vi "字符串解包.vi"(10 "输入数据":string, 11 "初始化缓存":i32[][](array[numeric])) -> (2 "解析后数据":i32[][](array[numeric]))   [LabVIEW 2020]
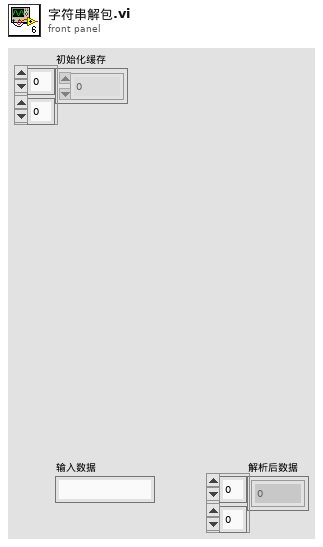
[diagram p1: front panel]
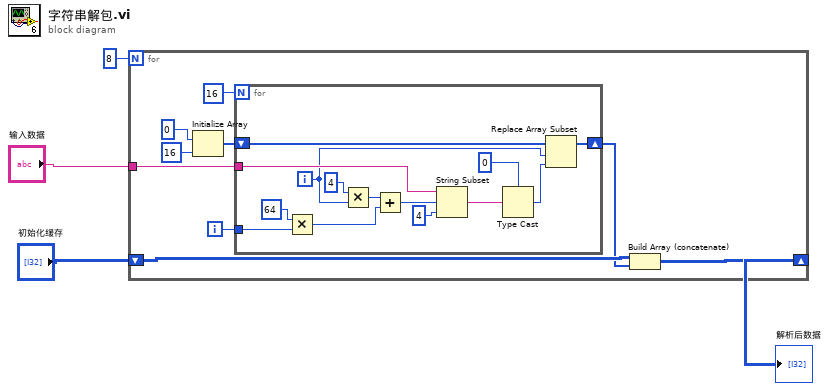
[diagram p0: block diagram]
diagram:
  n1 = for {
    N: u16 8 -> [_]
    tunnel: "输入数据" -> [w13]
    shift-right: [w6] -> w4
    shift-left: "初始化缓存" -> [w7]
    i -> [w8]
    n2 = Initialize Array(0, 16) -> (w9:i32[])
    n3 = for {
      N: i8 16 -> [_]
      tunnel: w13 -> [w25]
      tunnel: w8 -> [w21]
      shift-right: [w14] -> w5
      shift-left: w9 -> [w15]
      i -> [w16]
      n4 = Multiply(x=i8 64, y=w21) -> (x*y=w20:i32)
      n5 = Multiply(x=i8 4, y=w16) -> (x*y=w18:i32)
      n6 = Add(x=w18, y=w20) -> (x+y=w19:i32)
      n7 = String Subset(string=w25, offset (0)=w19, length (rest)=i8 4) -> (substring=w27:string)
      n8 = Type Cast(type=0, x=w27) -> (*(type *) &x=w17:i32)
      n9 = Replace Array Subset(array=w15, new element=w17, index=w16) -> (w14:i32[])
    }
    n10 = Build Array (concatenate)(w7, w5) -> (w6:i32[][])
  }
  "解析后数据" <- w4
